vi "RTS Single CMD.vi"(8 "error in (no error)":errorcluster, 10 "String":string, 11 "Modbus Master in":refnum<class "Modbus Master.lvclass">) -> (0 "error out":errorcluster, 3 "Modbus Master out":refnum<class "Modbus Master.lvclass">)   [LabVIEW 2016]
uses:
  <vilib>/NI/Modbus Library/API/Master/Modbus Master.lvclass
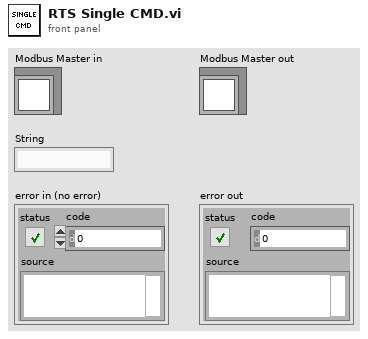
[diagram p1: front panel]
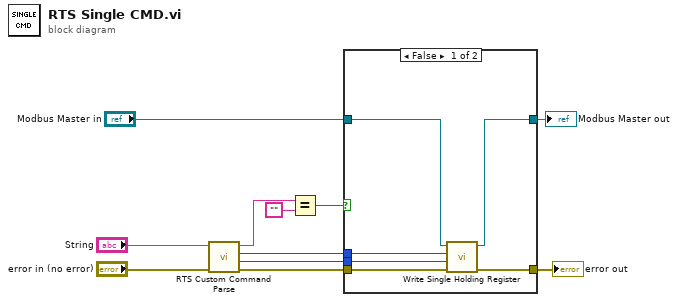
[diagram p0: block diagram]
diagram:
  n1 = call "RTS Custom Command Parse.vi"("Error In"="error in (no error)", "Input String"="String") -> ("Error Out"=w11:errorcluster, "Register to Write"=w8:i32, "Address"=w9:i32, "Clean Input String"=w7:string)  [unwired: 6 in]
  n2 = Equal?(x=w7, y="") -> (x = y?=w5:bool)
  n3 = case shown="False" w5 {
    tunnel: "Modbus Master in" -> [w17 w18]
    tunnel: [w16 w18] -> w2
    tunnel: w11 -> [w15 w19]
    tunnel: [w14 w19] -> w3
    tunnel: w8 -> [w13 _]
    tunnel: w9 -> [w12 _]
    frame False {
      n4 = call-dynamic "Write Single Holding Register.vi"("error in"=w15, "register to write"=w13, "address"=w12, "Modbus master in"=w17) -> ("error out"=w14:errorcluster, "Modbus master out"=w16:refnum<class "Modbus Master.lvclass">)  [unwired: 6 in]
    }
    frame True {
    }
  }
  "error out" <- w3
  "Modbus Master out" <- w2
